vi "HCC Search For UnUsed Stations.vi"(8 "Error In":errorcluster, 11 "Find Programs Named":string) -> (0 "Error Out":errorcluster, 1 "Name List":string[](array[string]), 2 "Array":i32[](array[numeric]), 3 "IDs 2":u32[](array[numeric]), 4 "Program Found!":bool)   [LabVIEW 2016]
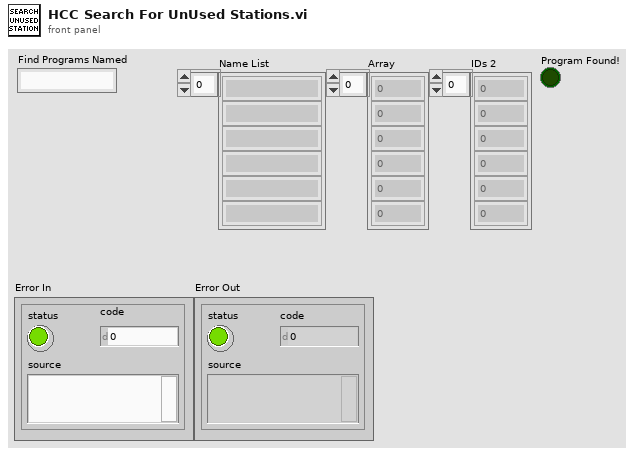
[diagram p1: front panel]
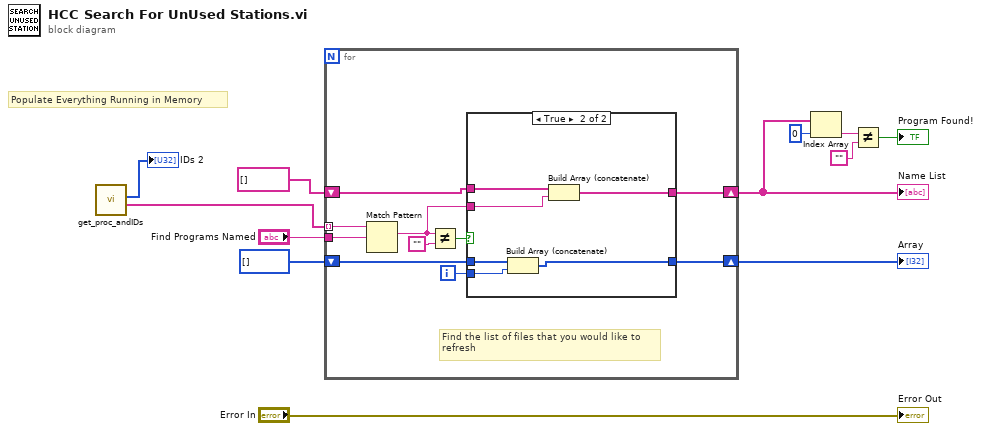
[diagram p0: block diagram]
diagram:
  # "Populate Everything Running in Memory"
  n1 = call "get_proc_andIDs.vi"() -> ("procese"=w9:string[], "IDs 2"=→"IDs 2":u32[])  [unwired: 10 out]
  n2 = for {
    tunnel: w9 -> [w18] mode=indexing
    shift-right: [w20] -> w11
    shift-left: i32[] [] -> [w21]
    tunnel: "Find Programs Named" -> [w17]
    shift-right: [w13] -> w6
    shift-left: string[] [] -> [w15]
    i -> [w19]
    # "Find the list of files that you would like to\nrefresh"
    n3 = Match Pattern(string=w18, regular expression=w17) -> (match substring=w14:string)  [unwired: 1 in, 3 out]
    n4 = Not Equal?(x=w14, y="") -> (x != y?=w22:bool)
    n5 = case shown="True" w22 {
      tunnel: w21 -> [w24 w30]
      tunnel: [w24 w29] -> w20
      tunnel: w19 -> [_ w28]
      tunnel: w15 -> [w23 w27]
      tunnel: w14 -> [_ w26]
      tunnel: [w23 w25] -> w13
      frame False {
      }
      frame True {
        n6 = Build Array (concatenate)(w30, w28) -> (w29:i32[])
        n7 = Build Array (concatenate)(w27, w26) -> (w25:string[])
      }
    }
  }
  "Array" <- w11
  "Name List" <- w6
  n8 = Index Array(array=w6, index=0) -> (element=w4:string)
  n9 = Not Equal?(x=w4, y="") -> (x != y?=→"Program Found!":bool)
  "Error Out" <- "Error In"
